vi "Memory.Pointer.Bounds Check.Length.vi"(8 "error in (no error)":errorcluster, 10 "length":i64 format="%d bytes", 11 "Pointer in":refnum<class "Memory.Pointer.lvclass">) -> (0 "error out":errorcluster, 1 "length valid":bool, 2 "length out":i64 format="%d bytes", 3 "Pointer out":refnum<class "Memory.Pointer.lvclass">)   [LabVIEW 2016, in "LabVIEW Memory Manager.lvlib" / "Memory.Pointer.lvclass"]
uses:
  Memory.Pointer.lvclass
  Memory.Pointer.lvclass/Memory.Pointer.ctl
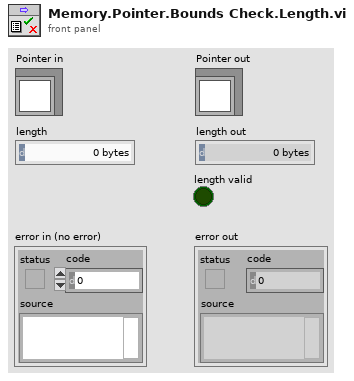
[diagram p1: front panel]
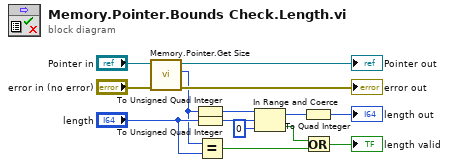
[diagram p0: block diagram]
diagram:
  n1 = call "Memory.Pointer.Get Size.vi"("error in (no error)"="error in (no error)", "Pointer in"="Pointer in") -> ("error out"=→"error out":errorcluster, "size"=w1:i64, "Pointer out"=→"Pointer out":refnum<class "Memory.Pointer.lvclass">)  [unwired: 7 in]
  n2 = To Unsigned Quad Integer(1:w1) -> (0:w9:u64)
  n3 = To Unsigned Quad Integer(1:"length") -> (0:w12:u64)
  n4 = Equal?(x=w1, y="length") -> (x = y?=w4:bool)
  n5 = In Range and Coerce(upper limit=w9, x=w12, lower limit=u64 0) -> (coerced(x)=w13:u64, In Range?=w3:bool)
  n6 = To Quad Integer(1:w13) -> (0:→"length out":i64)
  n7 = Or(x=w3, y=w4) -> (x .or. y?=→"length valid":bool)
